vi "read_attributes.vi"(8 "error in (no error)":errorcluster, 11 "MultinomialNB in":refnum<class "MultinomialNB.lvclass">) -> (0 "error out":errorcluster, 2 "attributes":T1, 3 "MultinomialNB out":refnum<class "MultinomialNB.lvclass">)   [LabVIEW 2020, in "MultinomialNB.lvclass"]
uses:
  MultinomialNB.lvclass
  Controls/multinomial_nb_attributes.ctl
  MultinomialNB.lvclass/MultinomialNB.ctl
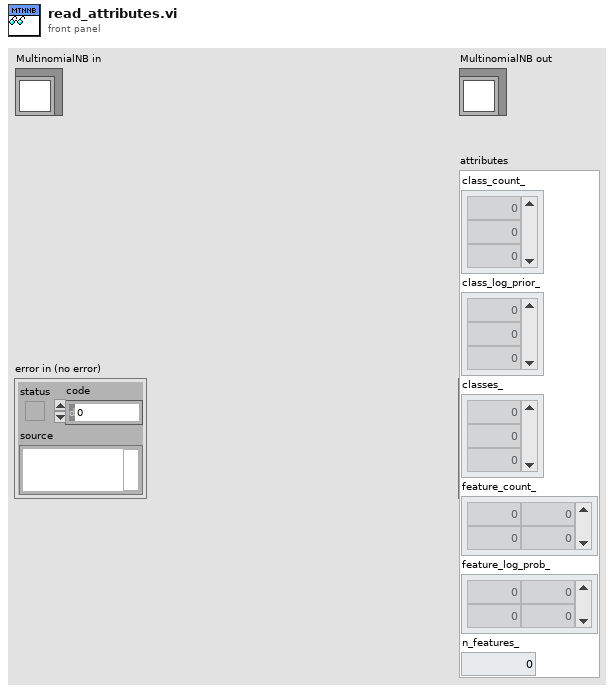
[diagram p1: front panel]
types:
  T1 = typedef "multinomial_nb_attributes.ctl" = cluster{"class_count_":dbl[], "class_log_prior_":dbl[], "classes_":dbl[], "feature_count_":dbl[][], "feature_log_prob_":dbl[][], "n_features_":dbl}
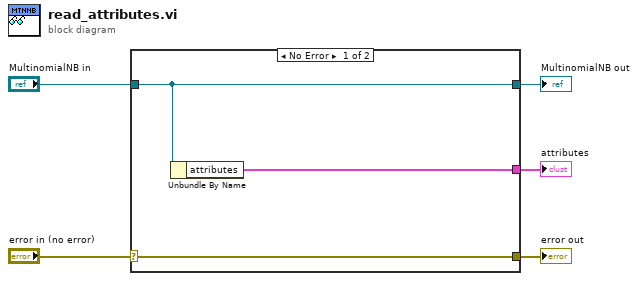
[diagram p0: block diagram]
diagram:
  n1 = case shown="No Error" "error in (no error)" {
    selector: "error in (no error)" -> [w8 w9]
    tunnel: [w8 w9] -> w4
    tunnel: [w7 w10] -> w2
    tunnel: "MultinomialNB in" -> [w7 w10]
    tunnel: [w6 _] -> w1
    frame No Error {
      n2 = Unbundle By Name(w7) -> ("attributes"=w6:T1)
    }
    frame Error {
    }
  }
  "error out" <- w4
  "MultinomialNB out" <- w2
  "attributes" <- w1
